vi "Parse GSV Sentence.vi"(8 "error in (no error)":errorcluster, 11 "GSV sentence":string) -> (0 "error out":errorcluster, 3 "GSV data":T1 {"satellite data"."data"."signal to noise ratio" min=0 max=99; "satellite data"."data"."azimuth (deg)" min=0 max=359; "satellite data"."data"."elevation (deg)" min=0 max=90; "number of satellites in view"."number of satellites" min=0; "sentence number"."number" min=0; "number of sentences for full data"."number of sentences" min=0})   [LabVIEW 2009]
doc: "Returns data contained in an NMEA sentence. You must manually select the polymorphic instance to use."
uses:
  typedefs/GSV Data.ctl
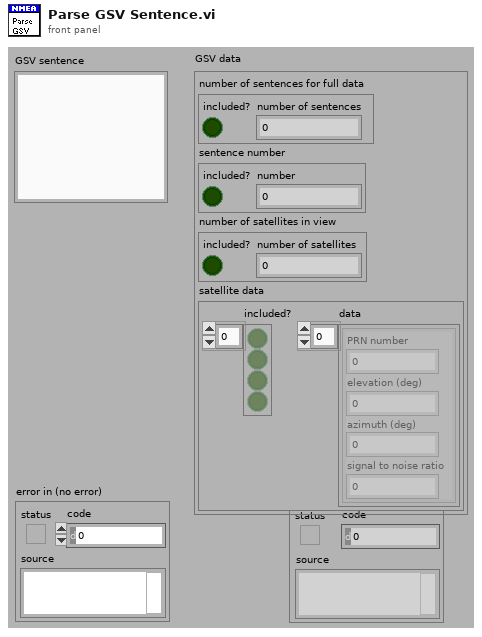
[diagram p1: front panel]
types:
  T1 = typedef "GSV Data.ctl" = cluster{"number of sentences for full data":cluster{"included?":bool, "number of sentences":i8}, "sentence number":cluster{"included?":bool, "number":i8}, "number of satellites in view":cluster{"included?":bool, "number of satellites":i8}, "satellite data":cluster{"included?":bool[], "data":cluster{"PRN number":i32, "elevation (deg)":i32, "azimuth (deg)":i32, "signal to noise ratio":i32}[]}}
  T2 = cluster{"Included?":bool[], "Satellite Data":cluster{"PRN Number":i32, "Elevation (deg)":i32, "Azimuth (deg)":i32, "Signal to Noise Ratio":i32}[]}
  T3 = cluster{"PRN Number":i32, "Elevation (deg)":i32, "Azimuth (deg)":i32, "Signal to Noise Ratio":i32}
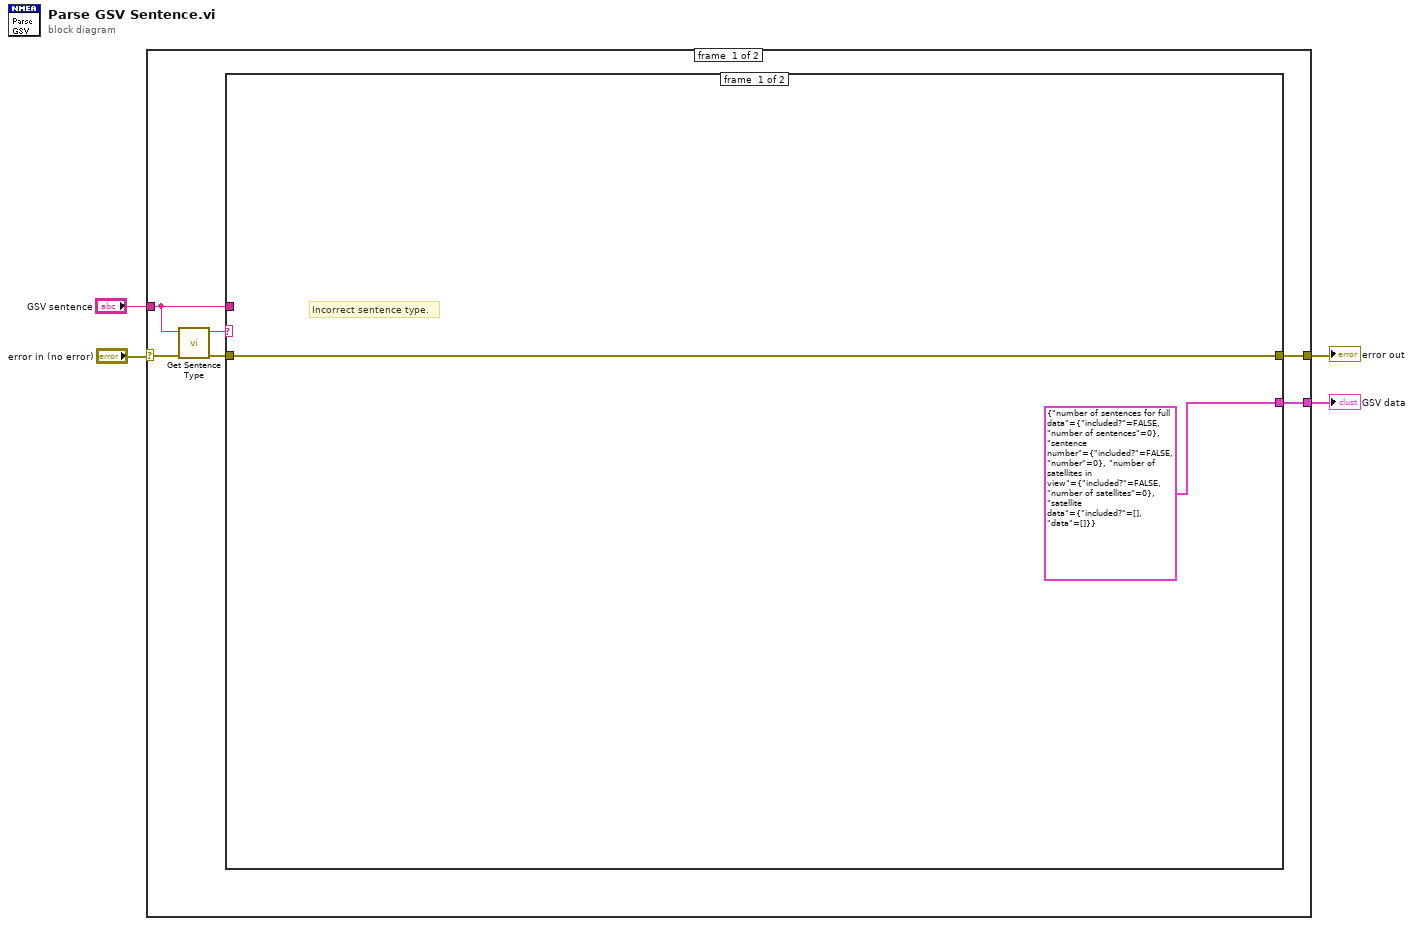
[diagram p0: block diagram]
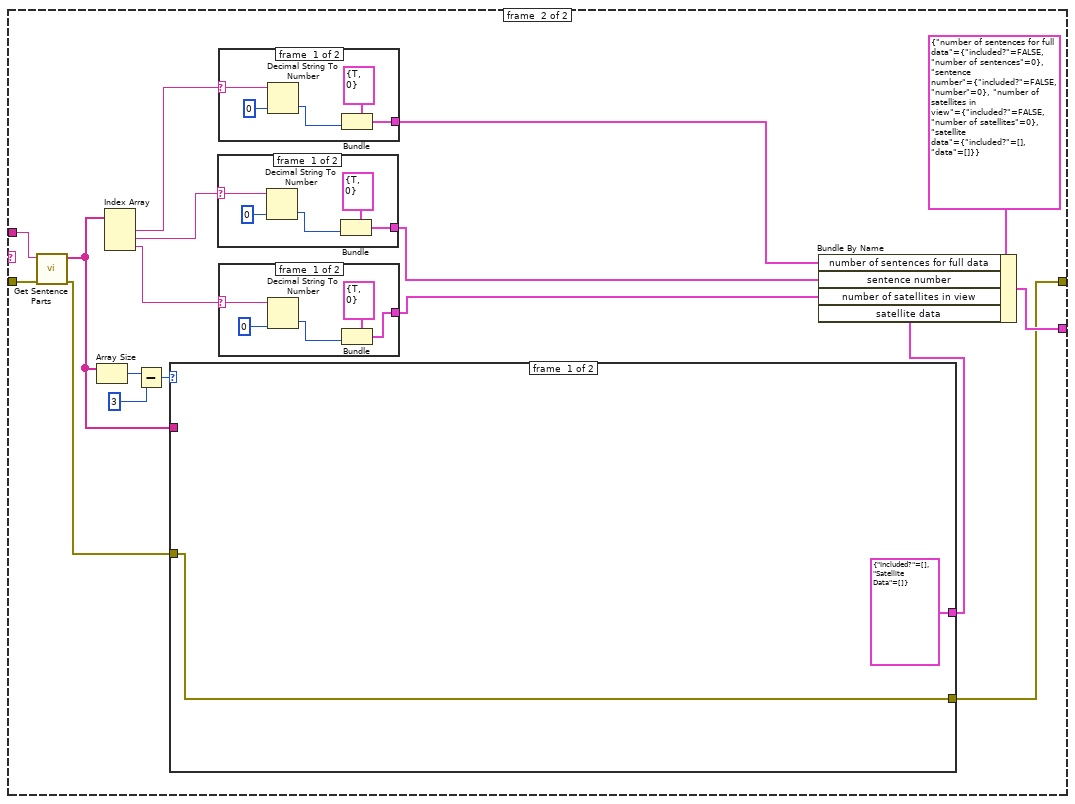
[diagram p2: hidden frame]
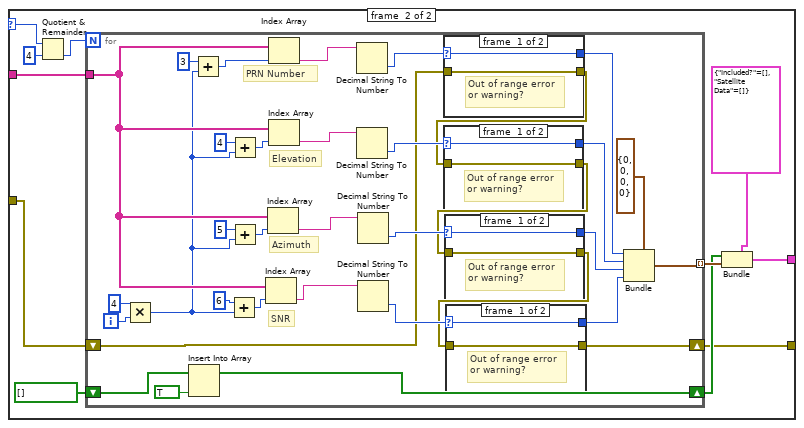
[diagram p3: hidden frame]
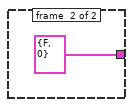
[diagram p8: hidden frame]
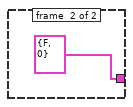
[diagram p9: hidden frame]
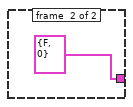
[diagram p10: hidden frame]
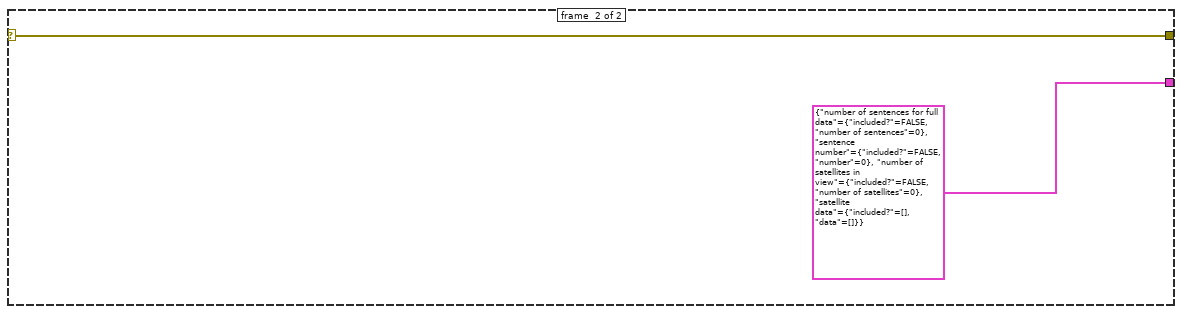
[diagram p11: hidden frame]
diagram:
  n1 = case shown="No Error" "error in (no error)" {
    selector: "error in (no error)" -> [w8 w112]
    tunnel: [w10 T1 {"number of sentences for full data"={"included?"=FALSE, "number of sentences"=0}, "sentence number"={"included?"=FALSE, "number"=0}, "number of satellites in view"={"included?"=FALSE, "number of satellites"=0}, "satellite data"={"included?"=[], "data"=[]}} ("GSV Data")] -> w4
    tunnel: [w9 w112] -> w3
    tunnel: "GSV sentence" -> [w6 _]
    frame #0 {
      n2 = call "Get Sentence Type.vi"("error in (no error)"=w8, "sentence"=w6) -> ("error out"=w7:errorcluster, "sentence type"=w5:string)  [unwired: 1 in, 7 out]
      n3 = case shown="\"GPGSV\"" w5 {
        tunnel: w7 -> [w11 w29]
        tunnel: w6 -> [_ w16]
        tunnel: [T1 {"number of sentences for full data"={"included?"=FALSE, "number of sentences"=0}, "sentence number"={"included?"=FALSE, "number"=0}, "number of satellites in view"={"included?"=FALSE, "number of satellites"=0}, "satellite data"={"included?"=[], "data"=[]}} ("GSV Data") w28] -> w10
        tunnel: [w11 w13] -> w9
        frame #0 {
          # "Incorrect sentence type."
        }
        frame #1 {
          n4 = call "Get Sentence Parts.vi"("error in (no error)"=w29, "sentence"=w16) -> ("error out"=w14:errorcluster, "sentence data"=w15:string[])  [unwired: 1 in, 7 out]
          n5 = Array Size(array=w15) -> (size(s)=w20:i32)
          n6 = Index Array(array=w15) -> (element #1=w26:string, element #2=w24:string, element #3=w23:string)  [unwired: 3 in]
          n7 = Subtract(x=w20, y=3) -> (x-y=w18:i32)
          n8 = case shown="1, Default" w18 {
            selector: w18 -> [_ w39]
            tunnel: w15 -> [_ w40]
            tunnel: [T2 {"Included?"=[], "Satellite Data"=[]} ("Satellite Data") w36] -> w17
            tunnel: w14 -> [w30 w33]
            tunnel: [w30 w32] -> w13
            frame #0 {
            }
            frame #1 {
              n9 = Quotient & Remainder(x=w39, y=4) -> (floor(x/y)=w41:i32)  [unwired: 1 out]
              n10 = for {
                N: w41 -> [_]
                tunnel: [w72] -> w38 mode=indexing
                tunnel: w40 -> [w68]
                shift-right: [w57] -> w34
                shift-left: bool[] [] ("Included?") -> [w59]
                shift-right: [w47] -> w32
                shift-left: w33 -> [w51]
                i -> [w70]
                # "SNR"
                # "Azimuth"
                # "Elevation"
                # "PRN Number"
                n11 = Multiply(x=4, y=w70) -> (x*y=w60:i32)
                n12 = Insert Into Array(array=w59, new element=TRUE ("new element/subarray")) -> (w57:bool[])  [unwired: 1 in]
                n13 = Add(x=3, y=w60) -> (x+y=w67:i32)
                n14 = Add(x=6, y=w60) -> (x+y=w61:i32)
                n15 = Add(x=4, y=w60) -> (x+y=w65:i32)
                n16 = Add(x=5, y=w60) -> (x+y=w63:i32)
                n17 = Index Array(array=w68, index=w61) -> (element=w73:string)
                n18 = Index Array(array=w68, index=w63) -> (element=w74:string)
                n19 = Index Array(array=w68, index=w67) -> (element=w76:string)
                n20 = Index Array(array=w68, index=w65) -> (element=w75:string)
                n21 = Decimal String To Number(string=w76) -> (number=w55:i32)  [unwired: 2 in, 1 out]
                n22 = Decimal String To Number(string=w75) -> (number=w54:i32)  [unwired: 2 in, 1 out]
                n23 = Decimal String To Number(string=w74) -> (number=w53:i32)  [unwired: 3 out]
                n24 = Decimal String To Number(string=w73) -> (number=w52:i32)  [unwired: 2 in, 1 out]
                n25 = case shown="Default" w55 {
                  selector: w55 -> [w89 w91]
                  tunnel: w51 -> [w90 w92]
                  tunnel: [w90 w92] -> w50
                  tunnel: [w89 w91] -> w46
                  frame #0 {
                    # "Out of range error\nor warning?"
                  }
                  frame #1 {
                    # "Valid range"
                  }
                }
                n26 = case shown="Default" w54 {
                  selector: w54 -> [w85 w87]
                  tunnel: w50 -> [w86 w88]
                  tunnel: [w86 w88] -> w49
                  tunnel: [w85 w87] -> w45
                  frame #0 {
                    # "Out of range error\nor warning?"
                  }
                  frame #1 {
                    # "Valid range"
                  }
                }
                n27 = case shown="Default" w53 {
                  selector: w53 -> [w81 w83]
                  tunnel: w49 -> [w82 w84]
                  tunnel: [w82 w84] -> w48
                  tunnel: [w81 w83] -> w44
                  frame #0 {
                    # "Out of range error\nor warning?"
                  }
                  frame #1 {
                    # "Valid range"
                  }
                }
                n28 = case shown="Default" w52 {
                  selector: w52 -> [w77 w79]
                  tunnel: w48 -> [w78 w80]
                  tunnel: [w78 w80] -> w47
                  tunnel: [w77 w79] -> w43
                  frame #0 {
                    # "Out of range error\nor warning?"
                  }
                  frame #1 {
                    # "Valid range"
                  }
                }
                n29 = Bundle(cluster=T3 {"PRN Number"=0, "Elevation (deg)"=0, "Azimuth (deg)"=0, "Signal to Noise Ratio"=0} ("Satellite 1 Data"), "PRN Number"=w46, "Elevation (deg)"=w45, "Azimuth (deg)"=w44, "Signal to Noise Ratio"=w43) -> (w72:T3)
              }
              n30 = Bundle(cluster=T2 {"Included?"=[], "Satellite Data"=[]} ("Satellite Data"), "Included?"=w34, "Satellite Data"=w38) -> (w36:T2)
            }
          }
          n31 = case shown="\"False\", Default" w24 {
            selector: w24 -> [w103 _]
            tunnel: [w100 cluster{"Valid?":bool, "# of Sentences":i8} {"Valid?"=FALSE, "# of Sentences"=0} ("Number of Sentences for Full Data")] -> w22
            frame #0 {
              n32 = Decimal String To Number(string=w103, default (0L)=i8 0) -> (number=w101:i8)  [unwired: 2 out]
              n33 = Bundle(cluster=cluster{"Valid?":bool, "# of Sentences":i8} {"Valid?"=TRUE, "# of Sentences"=0} ("Number of Sentences for Full Data"), "# of Sentences"=w101) -> (w100:cluster{"Valid?":bool, "# of Sentences":i8})  [unwired: 1 out]
            }
            frame #1 {
            }
          }
          n34 = case shown="\"False\", Default" w26 {
            selector: w26 -> [w109 _]
            tunnel: [w106 cluster{"Valid?":bool, "# of Sentences":i8} {"Valid?"=FALSE, "# of Sentences"=0} ("Number of Sentences for Full Data")] -> w25
            frame #0 {
              n35 = Decimal String To Number(string=w109, default (0L)=i8 0) -> (number=w107:i8)  [unwired: 2 out]
              n36 = Bundle(cluster=cluster{"Valid?":bool, "# of Sentences":i8} {"Valid?"=TRUE, "# of Sentences"=0} ("Number of Sentences for Full Data"), "# of Sentences"=w107) -> (w106:cluster{"Valid?":bool, "# of Sentences":i8})  [unwired: 1 out]
            }
            frame #1 {
            }
          }
          n37 = case shown="\"False\", Default" w23 {
            selector: w23 -> [w97 _]
            tunnel: [w94 cluster{"Valid?":bool, "# of Sentences":i8} {"Valid?"=FALSE, "# of Sentences"=0} ("Number of Sentences for Full Data")] -> w21
            frame #0 {
              n38 = Decimal String To Number(string=w97, default (0L)=i8 0) -> (number=w95:i8)  [unwired: 2 out]
              n39 = Bundle(cluster=cluster{"Valid?":bool, "# of Sentences":i8} {"Valid?"=TRUE, "# of Sentences"=0} ("Number of Sentences for Full Data"), "# of Sentences"=w95) -> (w94:cluster{"Valid?":bool, "# of Sentences":i8})  [unwired: 1 out]
            }
            frame #1 {
            }
          }
          n40 = Bundle By Name(cluster=T1 {"number of sentences for full data"={"included?"=FALSE, "number of sentences"=0}, "sentence number"={"included?"=FALSE, "number"=0}, "number of satellites in view"={"included?"=FALSE, "number of satellites"=0}, "satellite data"={"included?"=[], "data"=[]}} ("GSV Data"), "number of sentences for full data"=w25, "sentence number"=w22, "number of satellites in view"=w21, "satellite data"=w17) -> (w28:T1)
        }
      }
    }
    frame #1 {
    }
  }
  "error out" <- w3
  "GSV data" <- w4
